vi "globalSetUp.vi"(8 "error in":errorcluster, 11 "Loopback in":refnum<class "Logging Loopback.lvclass">) -> (0 "error out":errorcluster, 3 "Loopback out":refnum<class "Logging Loopback.lvclass">)   [LabVIEW 2020, in "Logging Loopback.lvclass"]
uses:
  Logging Loopback.lvclass
  niveristand-custom-device-testing-tools/VeriStandTestUtilities/VeriStandTestUtilities.lvlib
  Scripting/Ballard MIL-STD-1553 Scripting.lvlib
  Shared/Initialization Method.ctl
  Shared/Device Parameters.ctl
  <vilib>/WebDAVClient/NI_WebDAV.lvlib
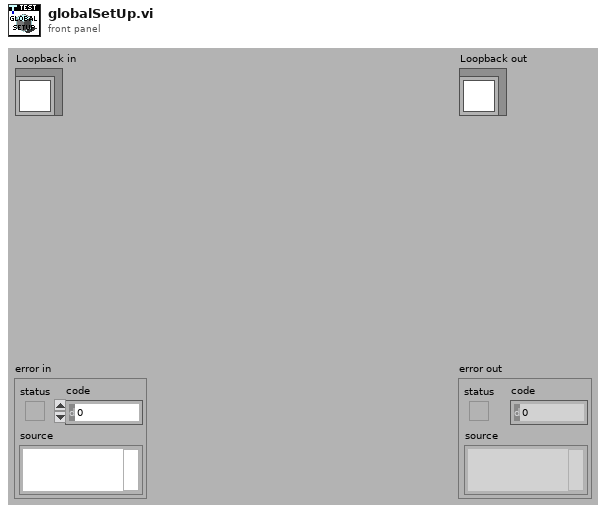
[diagram p1: front panel]
types:
  T1 = typedef "Device Parameters.ctl" = cluster{"initialization method":T2, "card number":i32, "PXI slot number":i32, "core number":i32}
  T2 = typedef "Initialization Method.ctl" = enum16{"PXI Slot Number", "Card Number"}
  T3 = typedef "Custom Device API.lvlib/Custom Device Item Ref.ctl" = u64
  T4 = typedef "NI_WebDAV.lvlib/SessionHandle.ctl" = refnum<k1>
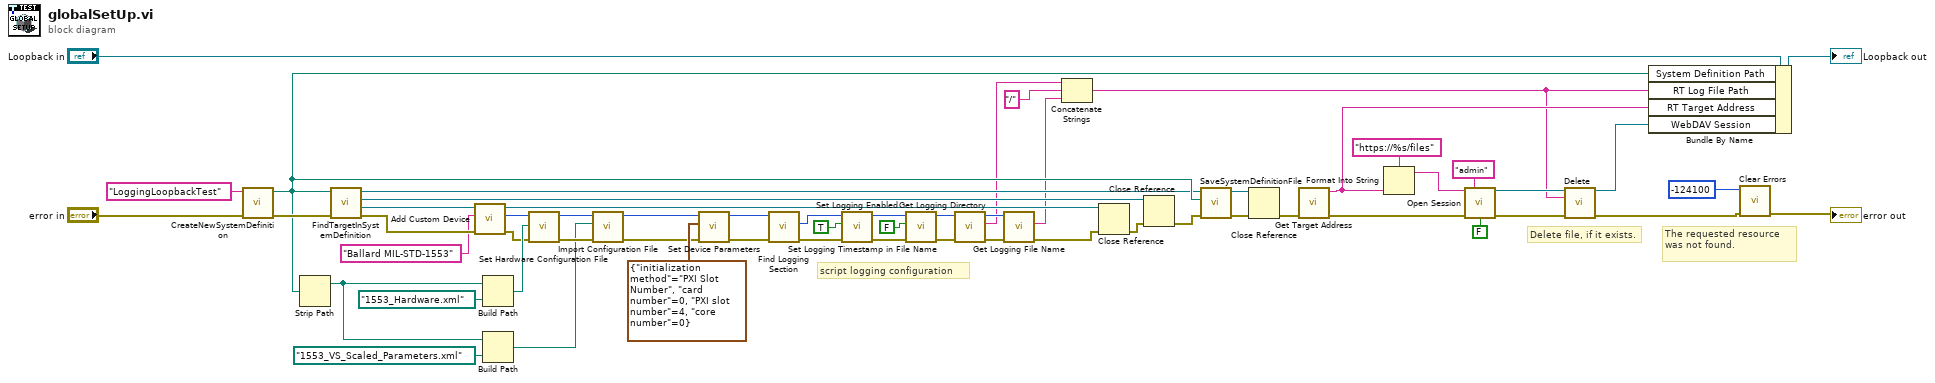
[diagram p0: block diagram]
diagram:
  # "script logging configuration"
  # "The requested resource was not found."
  # "Delete file, if it exists."
  n1 = call "CreateNewSystemDefinition.vi"("error in"="error in", "System Definition Name"="LoggingLoopbackTest") -> ("error out"=w58:errorcluster, "System Definition Path"=w57:path)  [unwired: 8 in]
  n2 = Strip Path(path=w57) -> (stripped path=w35:path)  [unwired: 1 out]
  n3 = call "FindTargetInSystemDefinition.vi"("error in"=w58, "system definition path"=w57) -> ("error out"=w49:errorcluster, "Target"=w43:refnum<k24>, "Root"=w44:refnum<k24>, "System Definition"=w42:refnum<k24>)  [unwired: 6 in]
  n4 = call "Add Custom Device.vi"("error in"=w49, "name"="Ballard MIL-STD-1553", "target in"=w43) -> ("error out"=w51:errorcluster, "Ballard MIL-STD 1553 custom device"=w50:T3, "target out"=w46:refnum<k24>)  [unwired: 6 in]
  n5 = Build Path(base path=w35, name or relative path=path "1553_Hardware.xml") -> (appended path=w53:path)
  n6 = Build Path(base path=w35, name or relative path=path "1553_VS_Scaled_Parameters.xml") -> (appended path=w34:path)
  n7 = call "Set Hardware Configuration File.vi"("error in"=w51, "hardware configuration file path"=w53, "Ballard MIL-STD 1553 custom device in"=w50) -> ("error out"=w38:errorcluster, "Ballard MIL-STD 1553 custom device out"=w37:T3)  [unwired: 7 in]
  n8 = call "Import Configuration File.vi"("error in"=w38, "parameters configuration file path"=w34, "Ballard MIL-STD 1553 custom device in"=w37) -> ("error out"=w32:errorcluster, "Ballard MIL-STD 1553 custom device out"=w31:T3)  [unwired: 7 in]
  n9 = call "Set Device Parameters.vi"("error in"=w32, "device parameters"=T1 {"initialization method"=enum."PXI Slot Number", "card number"=0, "PXI slot number"=4, "core number"=0}, "Ballard MIL-STD 1553 custom device in"=w31) -> ("error out"=w19:errorcluster, "Ballard MIL-STD 1553 custom device out"=w18:T3)  [unwired: 7 in]
  n10 = call "Find Logging Section.vi"("error in"=w19, "Ballard MIL-STD 1553 custom device in"=w18) -> ("error out"=w24:errorcluster, "logging"=w28:T3)  [unwired: 7 in, 1 out]
  n11 = call "Set Logging Enabled.vi"("error in"=w24, "logging enabled"=TRUE, "logging in"=w28) -> ("error out"=w23:errorcluster, "logging out"=w26:T3)  [unwired: 7 in]
  n12 = call "Set Logging Timestamp in File Name.vi"("error in"=w23, "timestamp in file name"=FALSE, "logging in"=w26) -> ("error out"=w21:errorcluster, "logging out"=w22:T3)  [unwired: 7 in]
  n13 = call "Get Logging Directory.vi"("error in"=w21, "logging in"=w22) -> ("error out"=w30:errorcluster, "directory"=w17:string, "logging out"=w29:T3)  [unwired: 7 in]
  n14 = call "Get Logging File Name.vi"("error in"=w30, "logging in"=w29) -> ("error out"=w20:errorcluster, "file name"=w15:string)  [unwired: 7 in, 1 out]
  n15 = Concatenate Strings(w17, "/" ("string"), w15) -> (w4:string)
  n16 = Close Reference(reference=w46, error in (no error)=w20) -> (error out=w47:errorcluster)
  n17 = Close Reference(reference=w44, error in (no error)=w47) -> (error out=w45:errorcluster)
  n18 = call "SaveSystemDefinitionFile.vi"("error in (no error)"=w45, "System Definition File in"=w57, "System Definition Reference in"=w42) -> ("error out"=w54:errorcluster, "System Definition Reference out"=w55:refnum<k24>)  [unwired: 7 in]
  n19 = Close Reference(reference=w55, error in (no error)=w54) -> (error out=w14:errorcluster)
  n20 = call "Get Target Address.vi"("error in"=w14) -> ("error out"=w9:errorcluster, "target address"=w8:string)  [unwired: 9 in]
  n21 = Format Into String(format string="https://%s/files" ("host uri prefix"), w8) -> (resulting string=w12:string)  [unwired: 2 in, 1 out]
  n22 = call <vilib>:"Open Session.vi"("host uri prefix"=w12, "username"="admin", "error in (no error)"=w9, "verify server?"=FALSE) -> ("session handle out"=w5:T4, "error out"=w7:errorcluster)  [unwired: 10 in]
  n23 = call <vilib>:"Delete.vi"("session handle"=w5, "relative uri"=w4, "error in (no error)"=w7) -> ("session handle out"=w6:T4, "error out"=w2:errorcluster)  [unwired: 11 in]
  n24 = Bundle By Name(cluster="Loopback in", "System Definition Path"=w57, "RT Log File Path"=w4, "RT Target Address"=w8, "WebDAV Session"=w6) -> (→"Loopback out":refnum<class "Logging Loopback.lvclass">)
  n25 = call <vilib>:"Clear Errors.vi"("error in (no error)"=w2, "specific error code to clear (0: all)"=-124100) -> ("error out"=→"error out":errorcluster)  [unwired: 4 in, 1 out]
